vi "TM620 Read Samp (SubVI).vi"(9 "channel":enum16{"Chan A", "Chan B", "Chan C", "Chan D"}(ring), 10 "semaphore TM620":T1, 11 "VISA Refnum in":refnum<visa-resource-name>) -> (2 "response out":string, 3 "VISA Refnum out":refnum<visa-resource-name>)   [LabVIEW 2019]
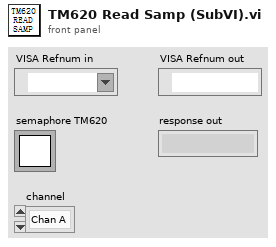
[diagram p1: front panel]
types:
  T1 = typedef "Semaphore RefNum" = refnum<k1>
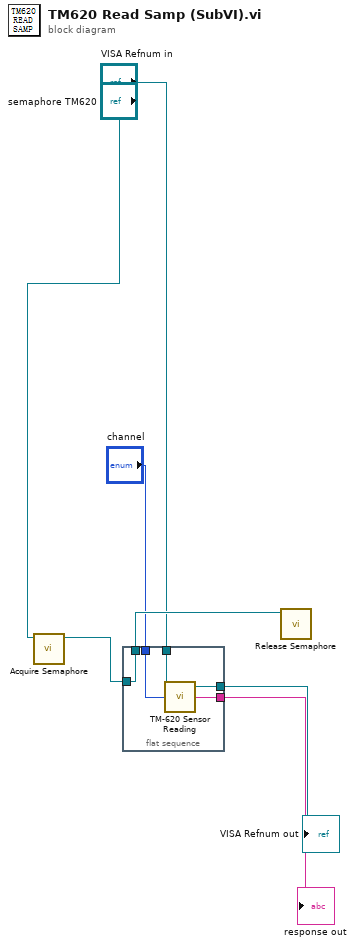
[diagram p0: block diagram]
diagram:
  n1 = call <vilib>:"Acquire Semaphore.vi"("semaphore"="semaphore TM620") -> ("semaphore out"=w5:T1)  [unwired: 4 in, 2 out]
  n2 = flat-sequence {
    tunnel: "VISA Refnum in" -> [w12]
    tunnel: "channel" -> [w11]
    tunnel: [w10] -> w3
    tunnel: [w9] -> w4
    tunnel: w5 -> [w8]
    tunnel: [w8] -> w6
    frame #0 {
      n3 = call "TM-620 Sensor Reading.vi"("channel"=w11, "VISA session"=w12) -> ("response out"=w9:string, "dup VISA session"=w10:refnum<visa-resource-name>)  [unwired: 1 in, 1 out]
    }
  }
  n4 = call <vilib>:"Release Semaphore.vi"("semaphore"=w6) -> ()  [unwired: 5 in, 2 out]
  "response out" <- w4
  "VISA Refnum out" <- w3
